vi "CData Unflatten String.vi"   [LabVIEW 2010]
uses:
  NXTFlattenXNode/CData Flatten XNode.xnode
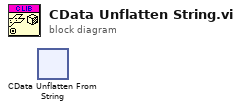
[diagram p0: block diagram]
diagram:
  n1 = xnode "CData Unflatten From String"() -> ()  [unwired: 3 in, 3 out]
